vi "MoveIn.vi"(8 "error in (no error)":errorcluster, 11 "reference in":refnum<class "DUT_Handler_Simple.lvclass">) -> (0 "error out":errorcluster, 1 "OK":bool, 3 "reference in":refnum<class "DUT_Handler_Simple.lvclass">)   [LabVIEW 2022 SP3, in "DUT_Handler_Simple.lvlib" / "DUT_Handler_Simple.lvclass"]
uses:
  DUT_Handler_Simple.lvclass
  Components/DUT_Handler_Base.lvlibp/Action.ctl
  Components/DUT_Handler_Base.lvlibp/EventData.ctl
  <vilib>/Utility/error.llb/Trim Whitespace One-Sided.vi
  Components/Barcode_Reader_Base.lvlibp/Barcode_Reader_Base.lvclass
  Components/DUT_Handler_Base.lvlibp/DUT_Handler_Base.lvclass
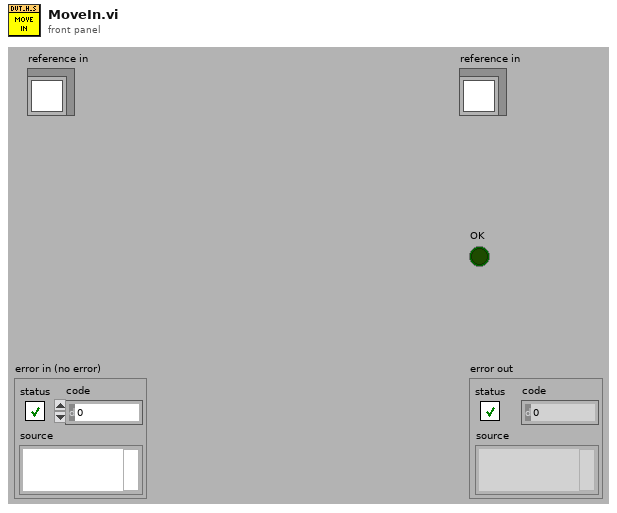
[diagram p1: front panel]
types:
  T1 = typedef "DUT_Handler_Base.lvlibp/DUT_Handler_Base.lvclass/EventData.ctl" = cluster{"Action":enum16{"Load", "Cancel", "MoveIn", "MoveOut", "Abort", "Msg", "Enabled", "Disabled", "Fault", "Shutdown"}, "SN":string, "BN":string, "DUT__ID":u32, "Message":string, "From":string, "To":string}
  T2 = typedef "DUT_Handler_Base.lvlibp/DUT_Handler_Base.lvclass/Action.ctl" = enum16{"Load", "Cancel", "MoveIn", "MoveOut", "Abort", "Msg", "Enabled", "Disabled", "Fault", "Shutdown"}
  T3 = typedef "DUT_Handler_Simple.lvlib/DUT_Handler_Simple.lvclass/ObjectAttributes.ctl" = cluster{"Config":T4, "event_data":T1, "Enabled":bool, "Barcode_Reader":refnum<class "Barcode_Reader_Base.lvclass">}
  T4 = typedef "DUT_Handler_Simple.lvlib/DUT_Handler_Simple.lvclass/Config.ctl" = cluster{"default":string}
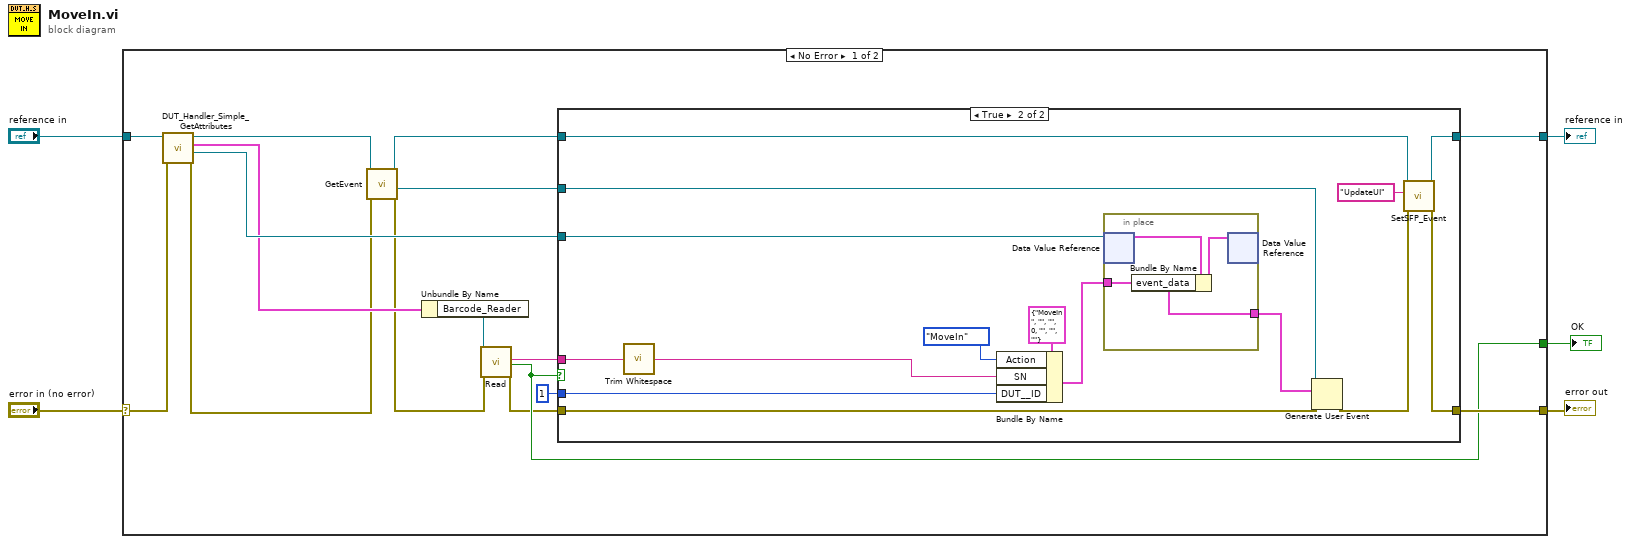
[diagram p0: block diagram]
diagram:
  n1 = case shown="No Error" "error in (no error)" {
    selector: "error in (no error)" -> [w21 w43]
    tunnel: [w16 w43] -> w4
    tunnel: [w17 w42] -> w2
    tunnel: "reference in" -> [w20 w42]
    tunnel: [w14 _] -> w1
    frame No Error {
      n2 = call "DUT_Handler_Simple_GetAttributes.vi"("error in (no error)"=w21, "reference in"=w20) -> ("error out"=w13:errorcluster, "DataRef"=w18:refnum<data-value>, "Data"=w15:T3, "reference out"=w19:refnum<class "DUT_Handler_Simple.lvclass">)  [unwired: 6 in]
      n3 = call-dynamic "GetEvent.vi"("error in (no error)"=w13, "reference in"=w19) -> ("error out"=w10:errorcluster, "DUT_Handler"=w12:refnum<user-event>, "reference in"=w11:refnum<class "DUT_Handler_Simple.lvclass">)  [unwired: 6 in]
      n4 = Unbundle By Name(w15) -> ("Barcode_Reader"=w8:refnum<class "Barcode_Reader_Base.lvclass">)
      n5 = call-dynamic "Read.vi"("reference in"=w8, "error in (no error)"=w10) -> ("Serial"=w7:string, "read Ok"=w14:bool, "error out"=w9:errorcluster)  [unwired: 14 in, 1 out]
      n6 = case shown="True" w14 {
        tunnel: w12 -> [_ w38]
        tunnel: w18 -> [_ w37]
        tunnel: w11 -> [w23 w36]
        tunnel: [w23 w35] -> w17
        tunnel: [w22 w34] -> w16
        tunnel: 1 ("DUT out") -> [_ w26]
        tunnel: w9 -> [w22 w27]
        tunnel: w7 -> [_ w25]
        frame False {
        }
        frame True {
          n7 = call <vilib>:"Trim Whitespace.vi"("string"=w25) -> ("trimmed string"=w24:string)  [unwired: 1 in]
          n8 = Bundle By Name(cluster=T1 {"Action"=enum."MoveIn", "SN"="", "BN"="", "DUT__ID"=0, "Message"="", "From"="", "To"=""} ("event_data"), "Action"=Action."MoveIn", "SN"=w24, "DUT__ID"=w26) -> (w30:T1)
          n9 = in-place {
            in-place-border: w30 -> [w39]
            in-place-border: [w39] -> w29
            n10 = in-place-dvr #1(w37) -> (w41:T3)  [unwired: 1 out]
            n11 = Bundle By Name(cluster=w41, "event_data"=w39) -> (w40:T3)
            n12 = in-place-dvr #1(w40) -> ()  [unwired: 2 out]
          }
          n13 = Generate User Event(user event=w38, event data cluster=w29, error in=w27) -> (error out=w33:errorcluster)  [unwired: 1 in, 1 out]
          n14 = call-dynamic "SetSFP_Event.vi"("error in (no error)"=w33, "msg"="UpdateUI", "reference in"=w36) -> ("error out"=w34:errorcluster, "reference out"=w35:refnum<class "DUT_Handler_Simple.lvclass">)  [unwired: 7 in]
        }
      }
    }
    frame Error {
    }
  }
  "error out" <- w4
  "reference in" <- w2
  "OK" <- w1
